vi "Add Category.vi"(8 "error in (no error)":errorcluster, 10 "Category Name":string, 11 "Budgetizer in":refnum<class "Budgetizer.lvclass">) -> (0 "error out":errorcluster, 2 "Anything Added?":bool, 3 "Budgetizer out":refnum<class "Budgetizer.lvclass">)   [LabVIEW 2018, in "Budgetizer.lvclass"]
uses:
  Budgetizer.lvclass
  Budgetizer.lvclass/Budgetizer.ctl
  database/Database.lvclass
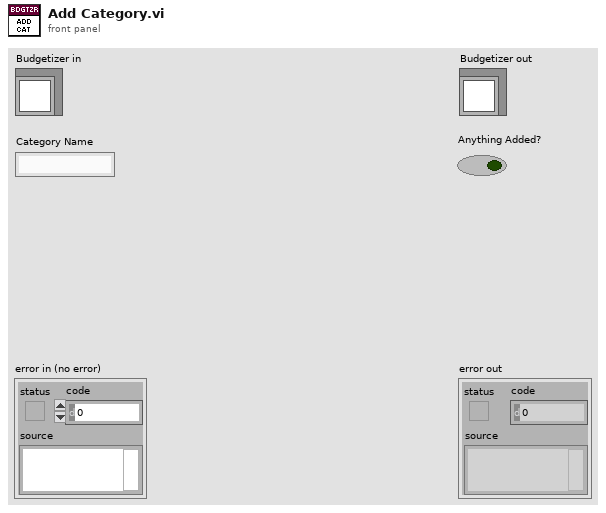
[diagram p1: front panel]
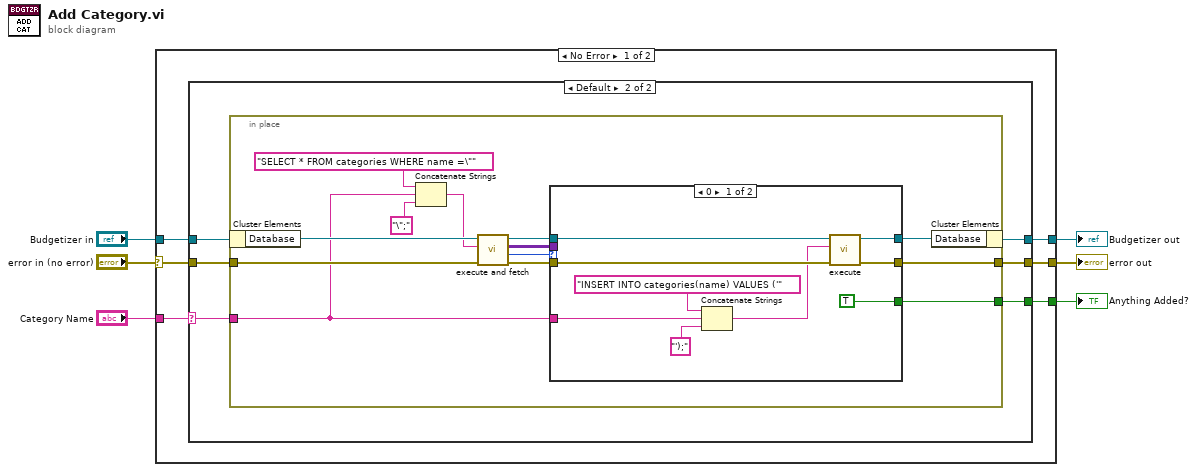
[diagram p0: block diagram]
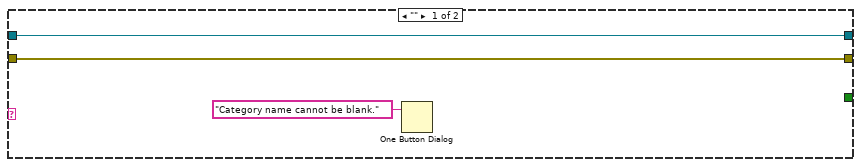
[diagram p2: hidden frame]
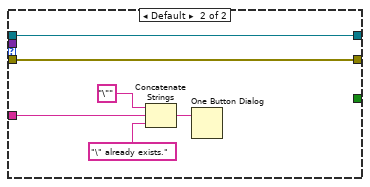
[diagram p3: hidden frame]
diagram:
  n1 = case shown="No Error" "error in (no error)" {
    selector: "error in (no error)" -> [w10 w51]
    tunnel: [w9 w51] -> w5
    tunnel: [w11 w50] -> w3
    tunnel: "Budgetizer in" -> [w12 w50]
    tunnel: "Category Name" -> [w8 _]
    tunnel: [w7 _] -> w1
    frame No Error {
      n2 = case shown="Default" w8 {
        selector: w8 -> [_ w17]
        tunnel: w12 -> [w15 w21]
        tunnel: [w15 w20] -> w11
        tunnel: w10 -> [w14 w19]
        tunnel: [w14 w18] -> w9
        tunnel: [_ w16] -> w7
        frame "" {
          n3 = One Button Dialog(message="Category name cannot be blank.") -> ()  [unwired: 1 in, 1 out]
        }
        frame Default {
          n4 = in-place {
            in-place-border: w17 -> [w23]
            in-place-border: w19 -> [w30]
            in-place-border: [w24] -> w18
            in-place-border: [w22] -> w16
            n5 = in-place-cluster #1(w21) -> ("Database"=w32:refnum<class "Database.lvclass">)
            n6 = Concatenate Strings("SELECT * FROM categories WHERE name =\"", w23, "\";") -> (w31:string)
            n7 = call "execute and fetch.vi"("error in (no error)"=w30, "SQL query"=w31, "Database in"=w32) -> ("error out"=w27:errorcluster, "Num records"=w28:i32, "recordset data"=w29:variant[][], "Database out"=w26:refnum<class "Database.lvclass">)  [unwired: 5 in]
            n8 = case shown="0" w28 {
              tunnel: w29 -> [_ _]
              tunnel: w27 -> [w42 w48]
              tunnel: w26 -> [w43 w49]
              tunnel: [w40 w49] -> w25
              tunnel: [w41 w48] -> w24
              tunnel: w23 -> [w37 w46]
              tunnel: [TRUE ("Anything Added?") _] -> w22
              frame 0 {
                n9 = Concatenate Strings("INSERT INTO categories(name) VALUES ('", w37, "');" ("string")) -> (w36:string)
                n10 = call "execute.vi"("error in (no error)"=w42, "SQL query"=w36, "Database in"=w43) -> ("error out"=w41:errorcluster, "Database out"=w40:refnum<class "Database.lvclass">)  [unwired: 7 in]
              }
              frame Default {
                n11 = Concatenate Strings("\"" ("string"), w46, "\" already exists." ("string")) -> (w45:string)
                n12 = One Button Dialog(message=w45) -> ()  [unwired: 1 in, 1 out]
              }
            }
            n13 = in-place-cluster #1("Database"=w25) -> (w20:refnum<class "Budgetizer.lvclass">)
          }
        }
      }
    }
    frame Error {
    }
  }
  "error out" <- w5
  "Budgetizer out" <- w3
  "Anything Added?" <- w1
